vi "probe_2_gaussians.vi"(3 "output control":T1, 4 "data":variant, 5 "X":dbl[](array[numeric]), 6 "a":dbl[](array[numeric])) -> (0 "error out":errorcluster, 1 "f'(X,a)":dbl[][](array[numeric]), 2 "f(X,a)":dbl[](array[numeric]))   [LabVIEW 2011]
uses:
  <vilib>/gmath/NumericalOptimization/LM_output select.ctl
  <vilib>/gmath/NI_Gmath.lvlib
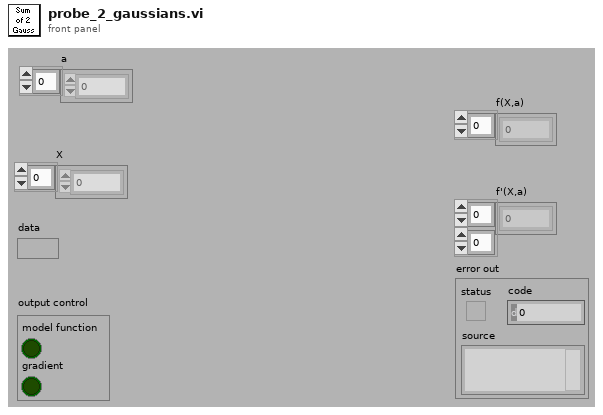
[diagram p1: front panel]
types:
  T1 = typedef "NI_Gmath.lvlib/LM_output select.ctl" = cluster{"model function":bool, "gradient":bool}
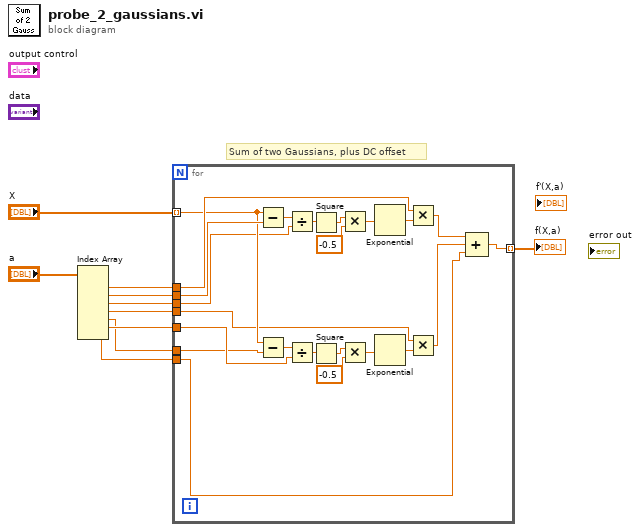
[diagram p0: block diagram]
diagram:
  # "Sum of two Gaussians, plus DC offset"
  n1 = Index Array(array="a") -> (element #1=w9:dbl, element #2=w4:dbl, element #3=w8:dbl, element #4=w7:dbl, element #5=w2:dbl, element #6=w3:dbl, element #7=w1:dbl)  [unwired: 7 in]
  n2 = for {
    tunnel: "X" -> [w27] mode=indexing
    tunnel: w9 -> [w31]
    tunnel: w4 -> [w33]
    tunnel: w8 -> [w19]
    tunnel: w7 -> [w26]
    tunnel: w3 -> [w18]
    tunnel: w1 -> [w12]
    tunnel: [w23] -> w6 mode=indexing
    tunnel: w2 -> [w11]
    n3 = Subtract(x=w27, y=w33) -> (x-y=w20:dbl)
    n4 = Subtract(x=w27, y=w11) -> (x-y=w17:dbl)
    n5 = Divide(x=w20, y=w19) -> (x/y=w32:dbl)
    n6 = Divide(x=w17, y=w18) -> (x/y=w28:dbl)
    n7 = Square(x=w32) -> (x^2=w16:dbl)
    n8 = Square(x=w28) -> (x^2=w15:dbl)
    n9 = Multiply(x=w16, y=-0.5) -> (x*y=w22:dbl)
    n10 = Multiply(x=w15, y=-0.5) -> (x*y=w21:dbl)
    n11 = Exponential(1:w22) -> (0:w30:dbl)
    n12 = Exponential(1:w21) -> (0:w29:dbl)
    n13 = Multiply(x=w31, y=w30) -> (x*y=w25:dbl)
    n14 = Multiply(x=w26, y=w29) -> (x*y=w24:dbl)
    n15 = Compound Arithmetic op=ADD(w25, w24, w12) -> (w23:dbl)
  }
  "f(X,a)" <- w6
